vi "CirceCalcSubVI.vi"(11 "Radius":dbl) -> (2 "Numeric 2":dbl, 3 "Numeric":dbl)   [LabVIEW 2018]
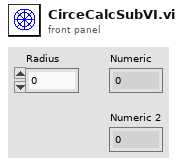
[diagram p1: front panel]
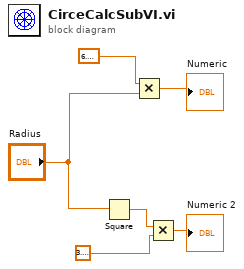
[diagram p0: block diagram]
diagram:
  n1 = Square(x="Radius") -> (x^2=w3:dbl)
  n2 = Multiply(x=6.283185307179586, y="Radius") -> (x*y=→"Numeric":dbl)
  n3 = Multiply(x=w3, y=3.141592653589793) -> (x*y=→"Numeric 2":dbl)
